vi "Initialize.vi"(0 "VISA resource name":refnum<visa-resource-name>, 5 "ID Query (T: Check)":bool=TRUE, 7 "Reset (T: Reset)":bool=TRUE, 11 "error in (no error)":errorcluster) -> (4 "VISA resource name out":refnum<visa-resource-name>, 15 "error out":errorcluster)   [LabVIEW 2013, in "Yokogawa.lvlib" / "Yokogawa PZ4000.lvlib"]
doc: "This VI passes the addressing information in the instrument decriptor to the Instr Open VI and returns the instrument ID. You can optionally reset the instrument by setting the front panel reset control. You must run this VI before using any of the instrument driver VIs for this instrument."
uses:
  Yokogawa PZ4000.lvlib
panel:
  # "Reset\nDon't Reset"
  # "Check\nDon't Check"
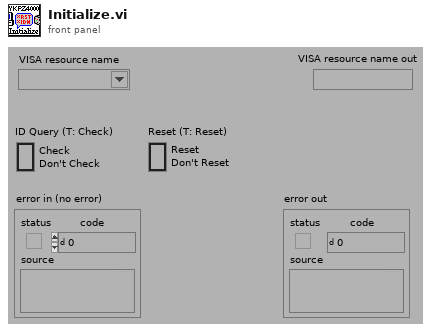
[diagram p1: front panel]
types:
  T1 = cluster{"status":bool, "Code":i32, "VI name":string}
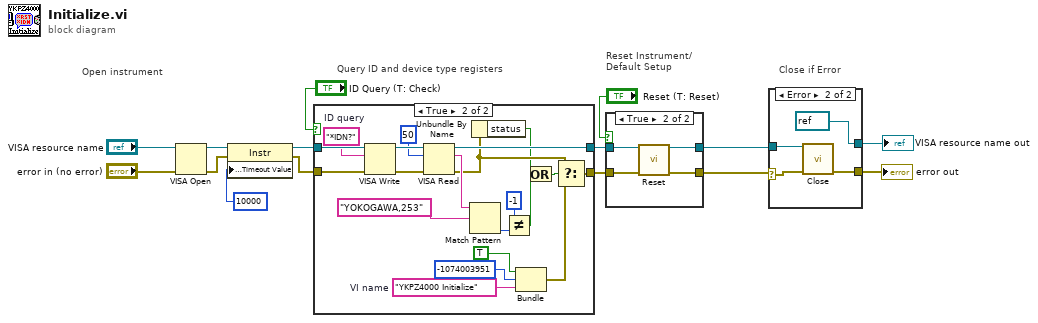
[diagram p0: block diagram]
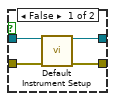
[diagram p3: hidden frame]
diagram:
  # "Reset Instrument/\nDefault Setup"
  # "Close if Error"
  # "Query ID and device type registers"
  # "Open instrument"
  n1 = VISA Open(error in (no error)="error in (no error)", VISA resource name="VISA resource name") -> (VISA resource name=w9:refnum<visa-resource-name>, error out=w8:errorcluster)  [unwired: 3 in]
  n2 = property class="Instr"(reference=w9, error in=w8, "General Settings:Timeout Value"=u32 10000 ("Tmo Value")) -> (reference out=w6:refnum<visa-resource-name>, error out=w5:errorcluster)
  n3 = case shown="True" "ID Query (T: Check)" {
    tunnel: [w16 w35] -> w14
    tunnel: [w17 w33] -> w15
    tunnel: w6 -> [w17 w31]
    tunnel: w5 -> [w16 w30]
    frame False {
    }
    frame True {
      w19 = "YKPZ4000 Initialize"  # VI name
      w29 = "*IDN?"  # ID query
      n4 = VISA Write(VISA resource name=w31, write buffer=w29, error in (no error)=w30) -> (VISA resource name out=w32:refnum<visa-resource-name>, error out=w37:errorcluster)  [unwired: 1 out]
      n5 = VISA Read(VISA resource name=w32, byte count=u32 50, error in (no error)=w37) -> (VISA resource name out=w33:refnum<visa-resource-name>, read buffer=w25:string, error out=w23:errorcluster)  [unwired: 1 out]
      n6 = Match Pattern(string=w25, regular expression="YOKOGAWA,253") -> (offset past match=w27:i32)  [unwired: 1 in, 3 out]
      n7 = Unbundle By Name(w23) -> ("status"=w21:bool)
      n8 = Not Equal?(x=-1, y=w27) -> (x != y?=w20:bool)
      n9 = Bundle(TRUE, "Code"=-1074003951, "VI name"=w19) -> (w34:cluster{bool, "Code":i32, "VI name":string})  [unwired: 1 in]
      n10 = Or(x=w21, y=w20) -> (x .or. y?=w22:bool)
      n11 = Select(t=w23, s=w22, f=w34) -> (s? t:f=w35:T1)
    }
  }
  n12 = case shown="True" "Reset (T: Reset)" {
    tunnel: w14 -> [w40 w45]
    tunnel: [w38 w44] -> w4
    tunnel: w15 -> [w41 w42]
    tunnel: [w39 w43] -> w3
    frame False {
      n13 = call "Default Instrument Setup.vi"("VISA resource name"=w41, "error in (no error)"=w40) -> ("VISA resource name out"=w39:refnum<visa-resource-name>, "error out"=w38:errorcluster)  [unwired: 12 in]
    }
    frame True {
      n14 = call "Reset.vi"("VISA resource name"=w42, "error in (no error)"=w45) -> ("VISA resource name out"=w43:refnum<visa-resource-name>, "error out"=w44:errorcluster)  [unwired: 12 in]
    }
  }
  n15 = case shown="Error" w4 {
    selector: w4 -> [w46 w51]
    tunnel: w3 -> [w47 w50]
    tunnel: [w46 w49] -> w1
    tunnel: [w47 refnum<visa-resource-name> refnum ("VISA resource name out")] -> w2
    frame No Error {
    }
    frame Error {
      n16 = call "Close.vi"("VISA resource name"=w50, "error in (no error)"=w51) -> ("error out"=w49:errorcluster)  [unwired: 13 in]
    }
  }
  "VISA resource name out" <- w2
  "error out" <- w1
